vi "test - loop references.vi"(8 "error in (no error)":errorcluster, 11 "TestCase in":refnum<class "csm-ini-variable-addon.lvclass">) -> (0 "error out":errorcluster, 3 "TestCase out":refnum<class "csm-ini-variable-addon.lvclass">)   [LabVIEW 2017, in "csm-ini-variable-addon.lvclass"]
uses:
  csm-ini-variable-addon.lvclass
  <vilib>/addons/_JKI Toolkits/VI Tester/TestCase.llb/TestCase.lvclass
  INI-Static-Variable-Support/INI-Static-Variable-Support.lvlib
  <userlib>/_NEVSTOP/Communicable State Machine(CSM)/addons/API-String-Arugments-Support/API String Arguments Support.lvlib
  C:/Program Files (x86)/National Instruments/LabVIEW 2017/vi.lib/addons/_JKI Toolkits/VI Tester/TestCase.llb/TestCase.lvclass
panel:
  out "String out 3":string
  out "String out 2":string
  out "String out":string
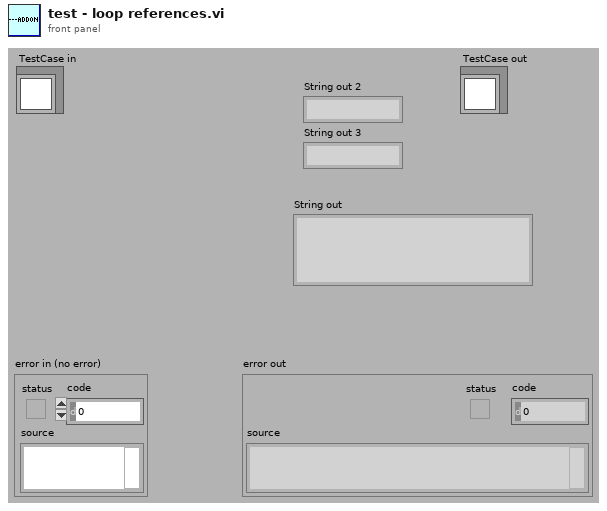
[diagram p1: front panel]
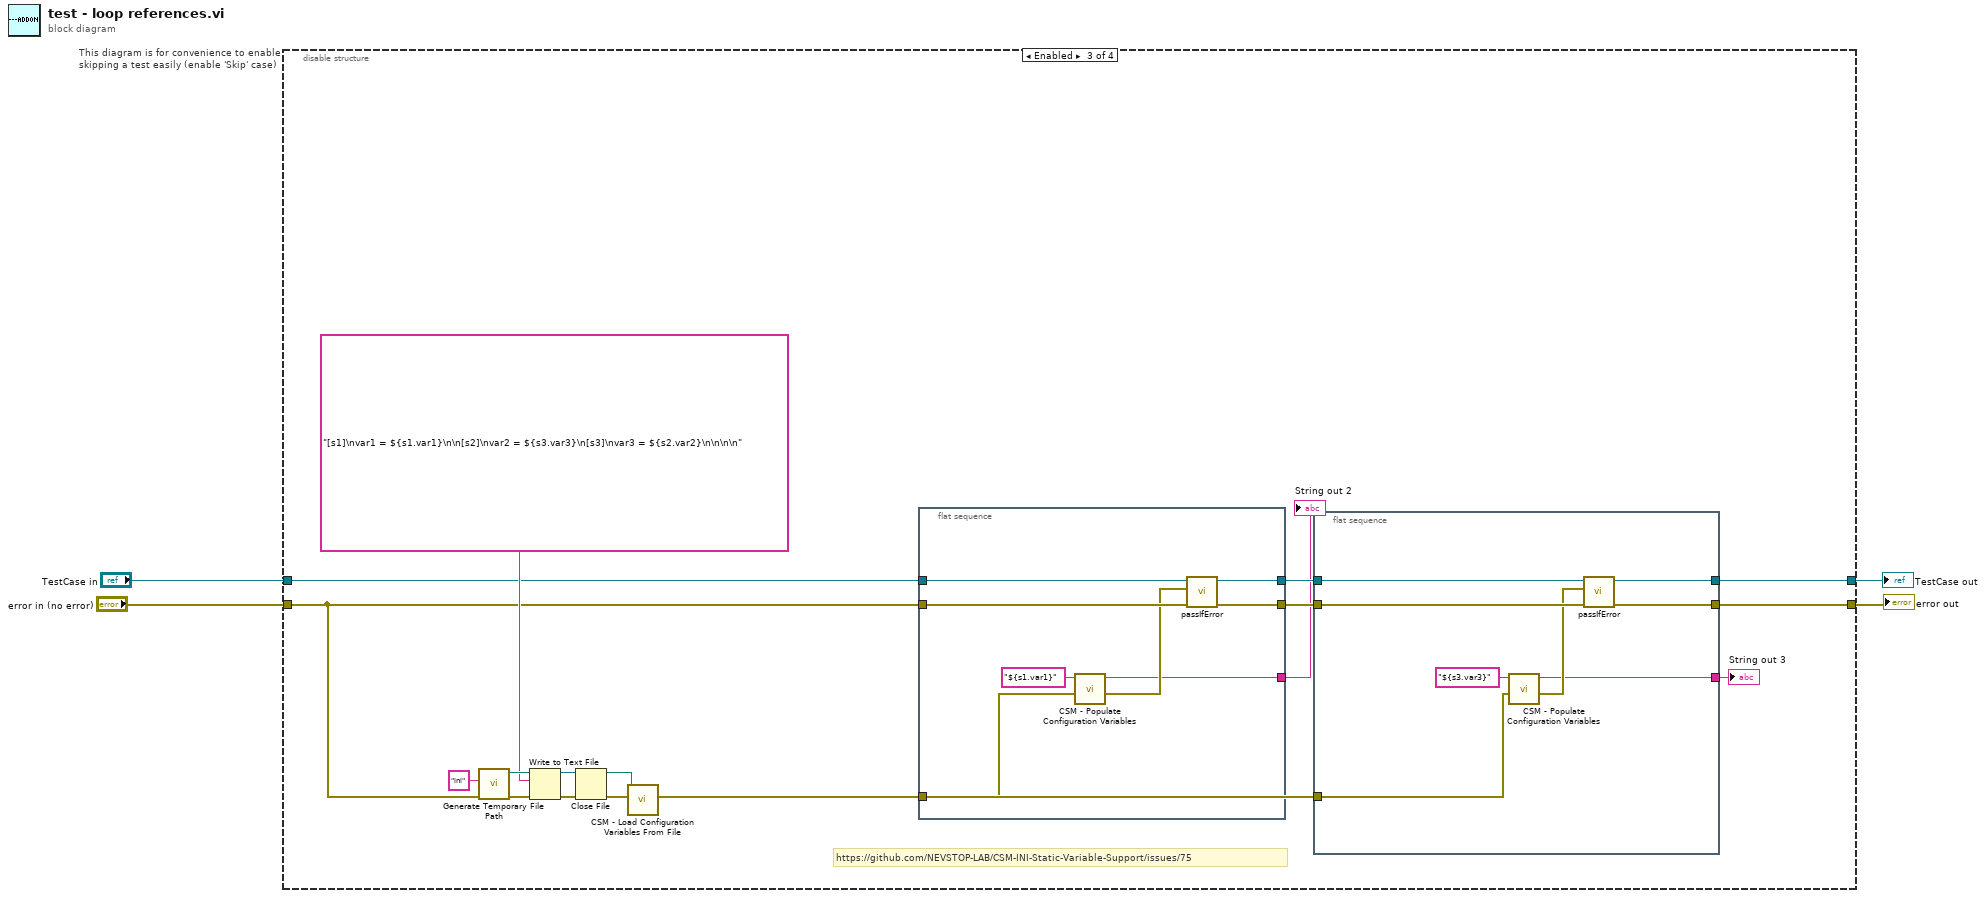
[diagram p0: block diagram]
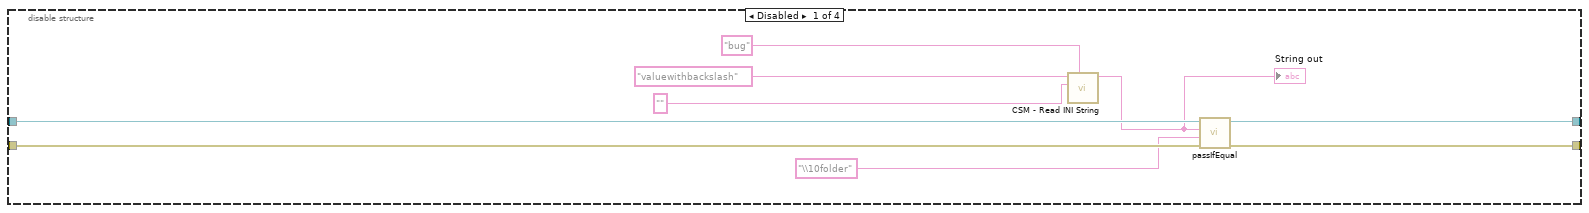
[diagram p2: hidden frame]
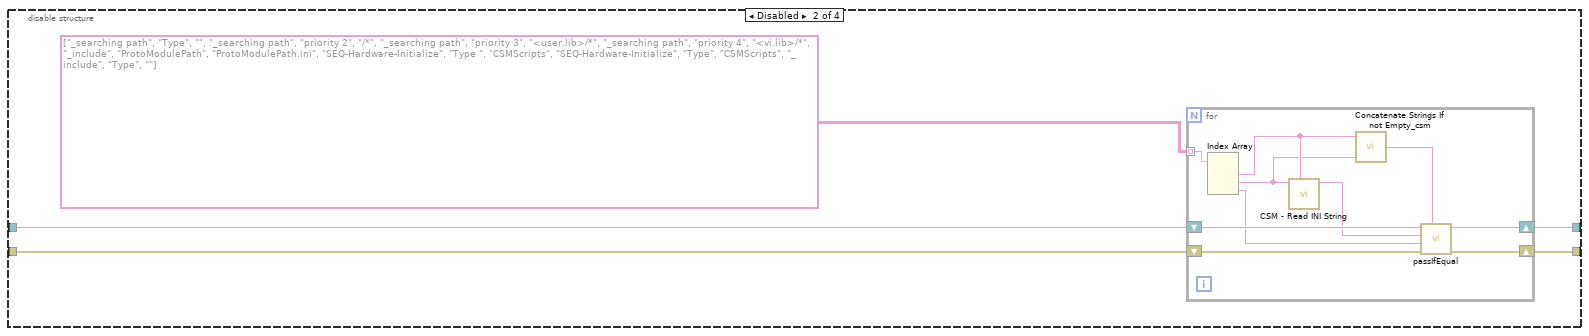
[diagram p3: hidden frame]
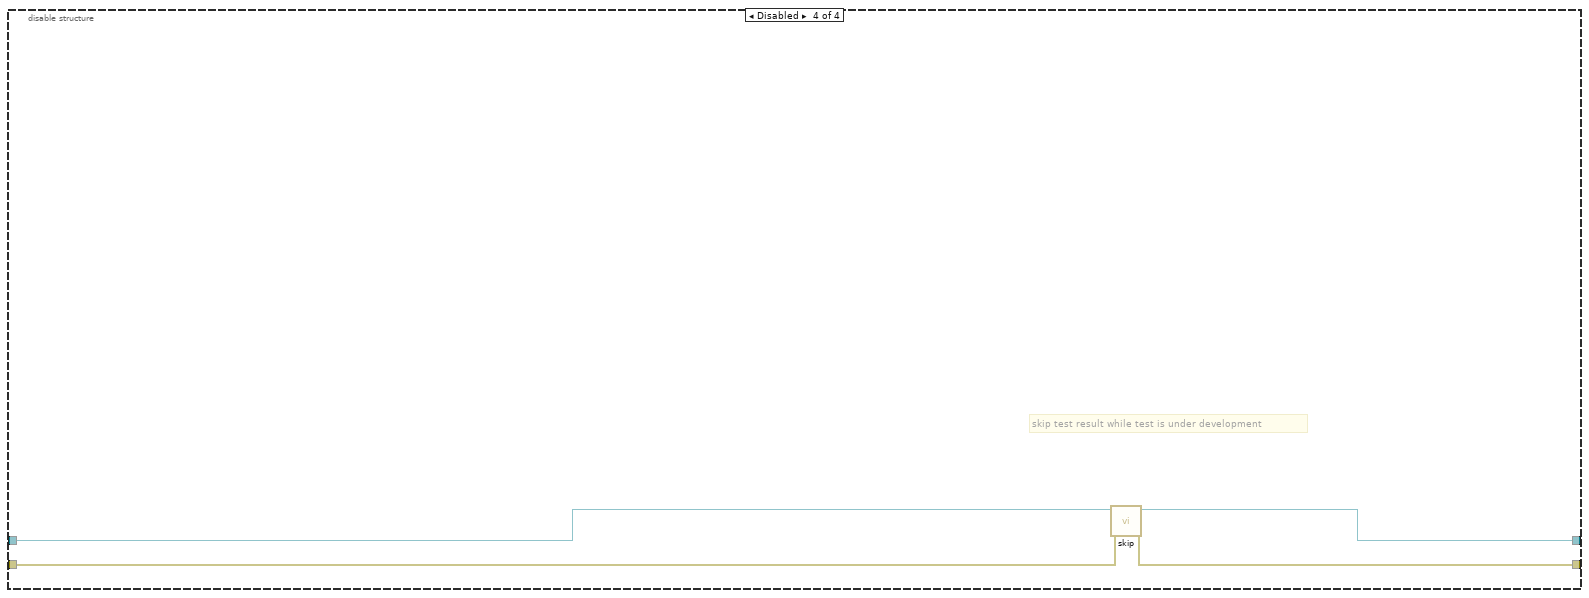
[diagram p4: hidden frame]
diagram:
  n1 = disable-structure "This diagram is for convenience to enable skipping a test easily (enable 'Skip' case)" shown="Enabled" {
    disable-tunnel: "TestCase in" -> [w10 w15 w37 w65]
    disable-tunnel: [w13 w18 w33 w63] -> w1
    disable-tunnel: [w12 w17 w34 w64] -> w3
    disable-tunnel: "error in (no error)" -> [w11 w16 w32 w62]
    frame Disabled {
      n2 = call "CSM - Read INI String.vi"("Section Name(\"\" as Default)"="bug" ("Section Name(\"\" as Default)"), ">> Default Value >>"="" ("String in"), "String in"="valuewithbackslash") -> ("String out"=w6:string)  [unwired: 4 in, 2 out]
      "String out" <- w6
      n3 = call-dynamic "passIfEqual.vi"("error in (no error)"=w11, "y"="\\10folder" ("String in"), "x"=w6, "TestCase in"=w10) -> ("error out"=w12:errorcluster, "TestCase out"=w13:refnum<class "csm-ini-variable-addon.lvclass">)  [unwired: 6 in]
    }
    frame Disabled {
      n4 = for {
        shift-right: [w27] -> w17
        shift-left: w16 -> [w26]
        shift-right: [w28] -> w18
        shift-left: w15 -> [w25]
        tunnel: string[][] [["_searching path", "Type", ""], ["_searching path", "priority 2", "/*"], ["_searching path", "priority 3", "<user.lib>/*"], ["_searching path", "priority 4", "<vi.lib>/*"], ["_include", "ProtoModulePath", "ProtoModulePath.ini"], ["SEQ-Hardware-Initialize", "Type ", "CSMScripts"], ["SEQ-Hardware-Initialize", "Type", "CSMScripts"], ["_include", "Type", ""]] -> [w23] mode=indexing
        n5 = Index Array(array=w23) -> (element #1=w20:string, element #2=w19:string, element #3=w22:string)  [unwired: 3 in]
        n6 = call "CSM - Read INI String.vi"("Section Name(\"\" as Default)"=w20, "String in"=w19) -> ("String out"=w24:string)  [unwired: 5 in, 2 out]
        n7 = call <userlib>:"Concatenate Strings If not Empty_csm.vi"("String"=w19, "prefix"=w20) -> ("result"=w21:string)  [unwired: 3 in]
        n8 = call-dynamic "passIfEqual.vi"("custom report message (\"\")"=w21, "error in (no error)"=w26, "y"=w22, "x"=w24, "TestCase in"=w25) -> ("error out"=w27:errorcluster, "TestCase out"=w28:refnum<class "csm-ini-variable-addon.lvclass">)  [unwired: 5 in]
      }
    }
    frame Enabled {
      # "https://github.com/NEVSTOP-LAB/CSM-INI-Static-Variable-Support/issues/75"
      n9 = call <vilib>:"Generate Temporary File Path.vi"("error in (no error)"=w32, "Temporary File Extension (tmp)"="ini") -> ("error out"=w45:errorcluster, "Unique Temporary File Path"=w42:path)  [unwired: 8 in]
      n10 = Write to Text File(file (use dialog)=w42, text="[s1]\nvar1 = ${s1.var1}\n\n[s2]\nvar2 = ${s3.var3}\n[s3]\nvar3 = ${s2.var2}\n\n\n\n", error in=w45) -> (refnum out=w41:refnum<file>, error out=w43:errorcluster)  [unwired: 1 in, 1 out]
      n11 = Close File(refnum=w41, error in=w43) -> (path=w38:path, error out=w40:errorcluster)
      n12 = call "CSM - Load Configuration Variables From File.vi"("error in (no error)"=w40, "Path"=w38) -> ("error out"=w31:errorcluster)  [unwired: 7 in]
      n13 = flat-sequence {
        tunnel: w37 -> [w61]
        tunnel: [w59] -> w36
        tunnel: [w58] -> w35
        tunnel: w32 -> [w57]
        tunnel: w31 -> [w55]
        tunnel: [w54] -> w30
        frame #0 {
          n14 = call "CSM - Populate Configuration Variables.vi"("error in (no error)"=w55, "String in"="${s1.var1}") -> ("error out"=w56:errorcluster, "String out"=w54:string)  [unwired: 6 in]
          n15 = call-dynamic "passIfError.vi"("error in (no error)"=w57, "error"=w56, "TestCase in"=w61) -> ("error out"=w58:errorcluster, "TestCase out"=w59:refnum<class "csm-ini-variable-addon.lvclass">)  [unwired: 7 in]
        }
      }
      n16 = flat-sequence {
        tunnel: w36 -> [w53]
        tunnel: w35 -> [w52]
        tunnel: [w51] -> w34
        tunnel: [w50] -> w33
        tunnel: w31 -> [w48]
        tunnel: [w46] -> w29
        frame #0 {
          n17 = call "CSM - Populate Configuration Variables.vi"("error in (no error)"=w48, "String in"="${s3.var3}") -> ("error out"=w47:errorcluster, "String out"=w46:string)  [unwired: 6 in]
          n18 = call-dynamic "passIfError.vi"("error in (no error)"=w52, "error"=w47, "TestCase in"=w53) -> ("error out"=w51:errorcluster, "TestCase out"=w50:refnum<class "csm-ini-variable-addon.lvclass">)  [unwired: 7 in]
        }
      }
      "String out 2" <- w30
      "String out 3" <- w29
    }
    frame Disabled {
      # "skip test result while test is under development"
      n19 = call <vilib>:"skip.vi"("error in (no error)"=w62, "TestCase in"=w65) -> ("error out"=w64:errorcluster, "TestCase out"=w63:refnum<class "csm-ini-variable-addon.lvclass">)  [unwired: 8 in]
    }
  }
  "error out" <- w3
  "TestCase out" <- w1
